vi "AppConfig.vi"(8 "error in (no error)":errorcluster, 11 "RingdownPlugin":refnum<class "EraPlugin.lvclass">=refnum) -> (0 "error out":errorcluster, 3 "RingdownPlugin out":refnum<class "EraPlugin.lvclass">)   [LabVIEW 2017, in "AppPlugins.lvlib" / "ERAPlugin.lvclass"]
uses:
  EraPlugin.lvclass
  ERAConfig.ctl
  Mode Estimation/COM_Preproc Parameters.ctl
  PublicAPI/TypeDef/RingdownConfig.ctl
  PublicAPI/TypeDef/ePhase.ctl
  EraPlugin.lvclass/EraPlugin.ctl
  Accessors/Read RingdownConfig.vi
  Accessors/Write RingdownConfig.vi
panel:
  in  "Phase":T1 items=["A", "B", "C"]
  out "RingdownConfig":T2={"Config"={"p_SysOdr"=2, "dThres"=0.1, "Preproc"={"order"=40, "f_lo"=0.1, "f_hi"=1.0, "R_down"=2}}, "V index"=0, "I index"=3, "PosSeq"=FALSE}
  in  "Cancel Button":bool
  in  "Save Button":bool
  in  "ERA Configuration":T3={"Threshold"=0.001, "Model Order"=2, "Preprocessing "={"order"=0, "f_lo"=0.0, "f_hi"=0.0, "R_down"=0}}
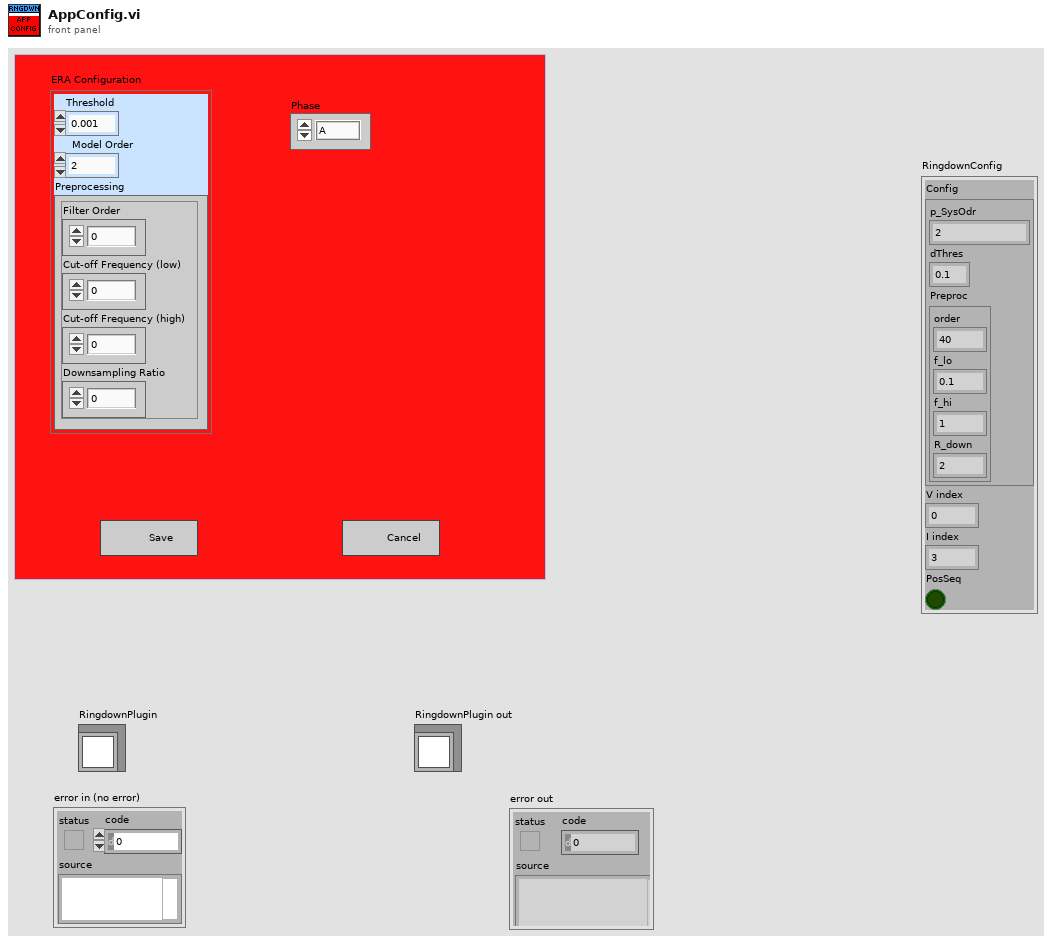
[diagram p1: front panel]
types:
  T1 = typedef "AppPlugins.lvlib/ERAPlugin.lvclass/ePhase.ctl" = u16
  T2 = typedef "AppPlugins.lvlib/ERAPlugin.lvclass/RingdownConfig.ctl" = cluster{"Config":cluster{"p_SysOdr":i32, "dThres":dbl, "Preproc":cluster{"order":i32, "f_lo":dbl, "f_hi":dbl, "R_down":i32}}, "V index":i32, "I index":i32, "PosSeq":bool}
  T3 = typedef "AppPlugins.lvlib/ERAPlugin.lvclass/ERAConfig.ctl" = cluster{"Threshold":dbl, "Model Order":i32, "Preprocessing ":T4}
  T4 = typedef "AppPlugins.lvlib/EraPlugin.lvclass/COM_Preproc Parameters.ctl" = cluster{"order":i32, "f_lo":dbl, "f_hi":dbl, "R_down":i32}
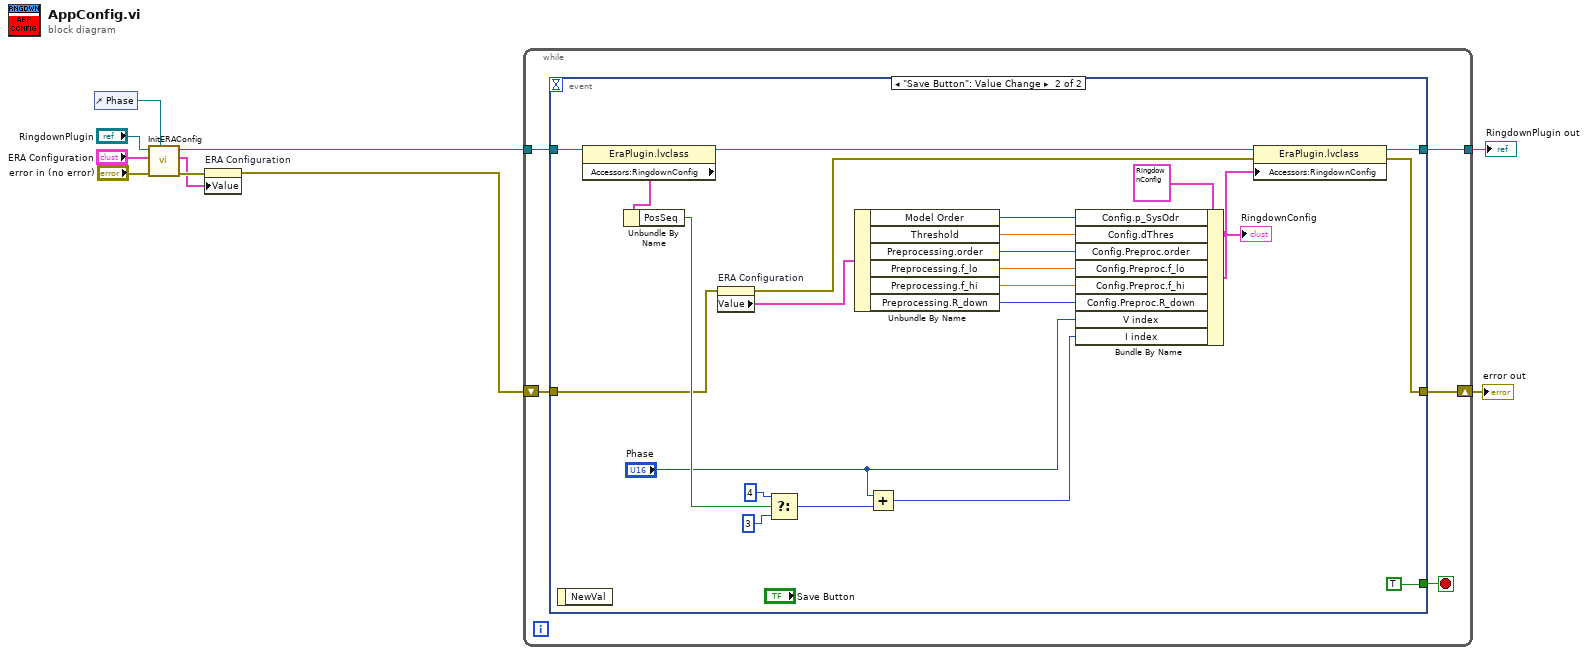
[diagram p0: block diagram]
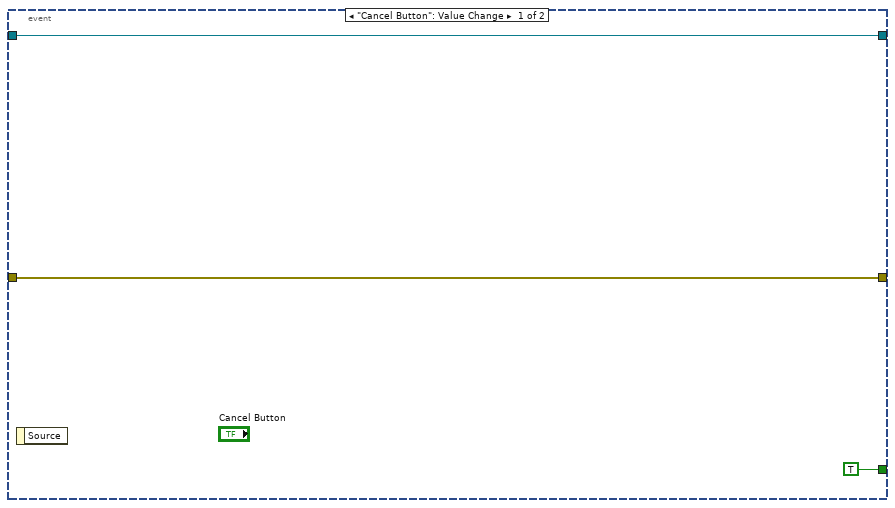
[diagram p2: hidden frame]
diagram:
  n1 = control-ref of="Phase"() -> (w2:refnum<vi>)
  n2 = call "InitERAConfig.vi"("Ring Refnum"=w2, "error in (no error)"="error in (no error)", "ERA Configuration"="ERA Configuration", "RingdownPlugin"="RingdownPlugin") -> ("error out"=w4:errorcluster, "ERA Configuration"=w3:T3, "RingdownPlugin"=w7:refnum<class "EraPlugin.lvclass">)  [unwired: 5 in]
  n3 = property on="ERA Configuration" class="Clust (strict)"(error in=w4, "Value"=w3) -> (error out=w1:errorcluster)  [unwired: 1 in, 1 out]
  n4 = while {
    shift-right: [w15] -> w10
    shift-left: w1 -> [w12]
    tunnel: w7 -> [w13]
    tunnel: [w14] -> w9
    stop <- w11 stop-if-true
    n5 = event shown="[1] \"Save Button\": Value Change" {
      selector: _ -> [_ _]
      dyn-events: _ -> [_ _]
      timeout: _ -> [_ _]
      tunnel: [w17 w41] -> w15
      tunnel: [w18 w40] -> w14
      tunnel: w13 -> [w18 w39]
      tunnel: w12 -> [w17 w25]
      tunnel: [TRUE TRUE] -> w11
      event "Cancel Button": Value Change {
        n6 = event-data() -> ()  [unwired: 1 in, 1 out]
      }
      event "Save Button": Value Change {
        n7 = event-data() -> ()  [unwired: 1 in, 1 out]
        n8 = property class="EraPlugin.lvclass"(reference=w39) -> (reference out=w31:refnum<class "EraPlugin.lvclass">, "Accessors:RingdownConfig"=w30:T2)  [unwired: 1 in, 1 out]
        n9 = Unbundle By Name(w30) -> ("PosSeq"=w29:bool)
        n10 = property on="ERA Configuration" class="Clust (strict)"(error in=w25) -> (error out=w33:errorcluster, "Value"=w34:T3)  [unwired: 1 in, 1 out]
        n11 = Select(t=u16 4 ("y"), s=w29, f=u16 3 ("y")) -> (s? t:f=w26:u16)
        n12 = Unbundle By Name(w34) -> ("Model Order"=w38:i32, "Threshold"=w36:dbl, "Preprocessing.order"=w24:i32, "Preprocessing.f_lo"=w23:dbl, "Preprocessing.f_hi"=w22:dbl, "Preprocessing.R_down"=w21:i32)
        n13 = Add(x="Phase", y=w26) -> (x+y=w19:T1)
        n14 = Bundle By Name(cluster=T2 {"Config"={"p_SysOdr"=-1, "dThres"=0.0, "Preproc"={"order"=1, "f_lo"=601.0, "f_hi"=10000.0, "R_down"=-1}}, "V index"=0, "I index"=1, "PosSeq"=FALSE} ("RingdownConfig"), "Config.p_SysOdr"=w38, "Config.dThres"=w36, "Config.Preproc.order"=w24, "Config.Preproc.f_lo"=w23, "Config.Preproc.f_hi"=w22, "Config.Preproc.R_down"=w21, "V index"="Phase", "I index"=w19) -> (w32:T2)
        "RingdownConfig" <- w32
        n15 = property class="EraPlugin.lvclass"(reference=w31, error in=w33, "Accessors:RingdownConfig"=w32) -> (reference out=w40:refnum<class "EraPlugin.lvclass">, error out=w41:errorcluster)
      }
    }
  }
  "error out" <- w10
  "RingdownPlugin out" <- w9
